vi "Turret_Homing.vi"(6 "Controller_Command":dbl, 7 "Turret_Motor_DefRef":T1={"DeviceStatus"={"status"=FALSE, "code"=0, "source"=""}, "Type"=enum."PWM", "PWM"={"PWM Channel"=enum."Invalid", "DeadBand"={"Name"="", "maxPositivePwm"=0, "minPositivePwm"=0, "centerPwm"=0, "maxNegativePwm"=0, "minNegativePwm"=0, "angularRange"=0}}, "CAN"={"Device Number"=0, "SetOutput VI Ref"=variant(enum8{"Percent VBus", "Current", "Speed", "Position", "Voltage"} enum."Percent VBus"), "GetOutput VI Ref"=variant(refnum<k1> refnum), "Enable VI Ref"=variant(dbl 12.0), "Disable VI Ref"=variant(enum8{"Percent VBus", "Speed", "Position", "Slave", "Unchanged / Invalid", "Voltage Compensation", "Current", "Motion Profile"} enum."Percent VBus"), "Data"=variant}, "Invert"=FALSE, "DIO PWM"={"PWM \"Enable\" Channel"=enum."Invalid", "DIOChannel"=enum."Invalid", "PWM Rate"=0.0}}, 8 "TurretManualHoming":bool, 9 "Reset":bool, 10 "Home_Position":dbl, 11 "MotorConfig":T6={"CAN Address"=0, "Invert"=FALSE, "InvertSensor"=FALSE, "Unit Conversion Factor"=0.0, "Brake Mode"=enum."Override to Brake", "Reverse Limt Switch Mode"=enum."Disabled", "Forward Limt Swith Mode"=enum."Disabled", "PWM Channel"=enum."Invalid", "Motor Controller Type"=enum."Talon SRX", "Peak Current (A)"=0, "Continuous Current (A)"=0, "Peak Duration (ms)"=0, "Current Limit Enable"=FALSE}) -> (1 "Motor_Output":dbl, 2 "Homing_State":T10, 3 "Turret_Motor_DefRef Out":T1={"DeviceStatus"={"status"=FALSE, "code"=0, "source"=""}, "Type"=enum."PWM", "PWM"={"PWM Channel"=enum."Invalid", "DeadBand"={"Name"="", "maxPositivePwm"=0, "minPositivePwm"=0, "centerPwm"=0, "maxNegativePwm"=0, "minNegativePwm"=0, "angularRange"=0}}, "CAN"={"Device Number"=0, "SetOutput VI Ref"=variant(enum8{"Percent VBus", "Current", "Speed", "Position", "Voltage"} enum."Percent VBus"), "GetOutput VI Ref"=variant(refnum<k1> refnum), "Enable VI Ref"=variant(dbl 12.0), "Disable VI Ref"=variant(enum8{"Percent VBus", "Speed", "Position", "Slave", "Unchanged / Invalid", "Voltage Compensation", "Current", "Motion Profile"} enum."Percent VBus"), "Data"=variant}, "Invert"=FALSE, "DIO PWM"={"PWM \"Enable\" Channel"=enum."Invalid", "DIOChannel"=enum."Invalid", "PWM Rate"=0.0}}, 5 "MotorConfigOut":T6={"CAN Address"=0, "Invert"=FALSE, "InvertSensor"=FALSE, "Unit Conversion Factor"=0.0, "Brake Mode"=enum."Override to Brake", "Reverse Limt Switch Mode"=enum."Disabled", "Forward Limt Swith Mode"=enum."Disabled", "PWM Channel"=enum."Invalid", "Motor Controller Type"=enum."Talon SRX", "Peak Current (A)"=0, "Continuous Current (A)"=0, "Peak Duration (ms)"=0, "Current Limit Enable"=FALSE})   [LabVIEW 2019]
uses:
  <vilib>/Rock Robotics/WPI/MotorControl/WPI_MotorControlDeviceRef.ctl
  <vilib>/Rock Robotics/WPI/MotorControl/WPI_MotorControlType.ctl
  <vilib>/Rock Robotics/SystemInterfaces/DIO/FPGA_DIOPWMChannel.ctl
  <vilib>/Rock Robotics/WPI/PWM/WPI_PWMDeadband.ctl
  <vilib>/Rock Robotics/SystemInterfaces/DIO/FPGA_DIOChannel.ctl
  ArgosLib/Config/ConfigComponents/TypeDefs/Config_Motor.ctl
  <vilib>/Rock Robotics/WPI/ThirdParty/Phoenix-LabVIEW/Motor Controller/Controls/CTRE_Phoenix_MotorControl_NeutralMode.ctl
  <vilib>/Rock Robotics/WPI/ThirdParty/Phoenix-LabVIEW/Motor Controller/Controls/CTRE_Phoenix_MotorControl_LimitSwitchNormal.ctl
  ArgosLib/Config/ConfigComponents/TypeDefs/Config_MotorCtrlType.ctl
  TypeDefs/Hood_Homing_State.ctl
  ArgosLib/Signal Processing/TypeDefs/EdgeDetector_Type.ctl
  <vilib>/Rock Robotics/WPI/ThirdParty/Phoenix-LabVIEW/Motor Controller/Controls/CTRE_Phoenix_MotorControl_FeedbackDevice.ctl
  TypeDefs/Read_or_Write.ctl
  584e72e6-e2ca-4219-9e99-eb915a757e0e.vi
  <vilib>/Rock Robotics/WPI/ThirdParty/Phoenix-LabVIEW/Motor Controller/Get/CTRE_Phoenix_MotorController_GetPulseWidthAll.vi
  <vilib>/Rock Robotics/WPI/ThirdParty/Phoenix-LabVIEW/Motor Controller/Get/CTRE_Phoenix_MotorController_GetSelectedSensorData.vi
  ArgosLib/ArgosLib.lvlib
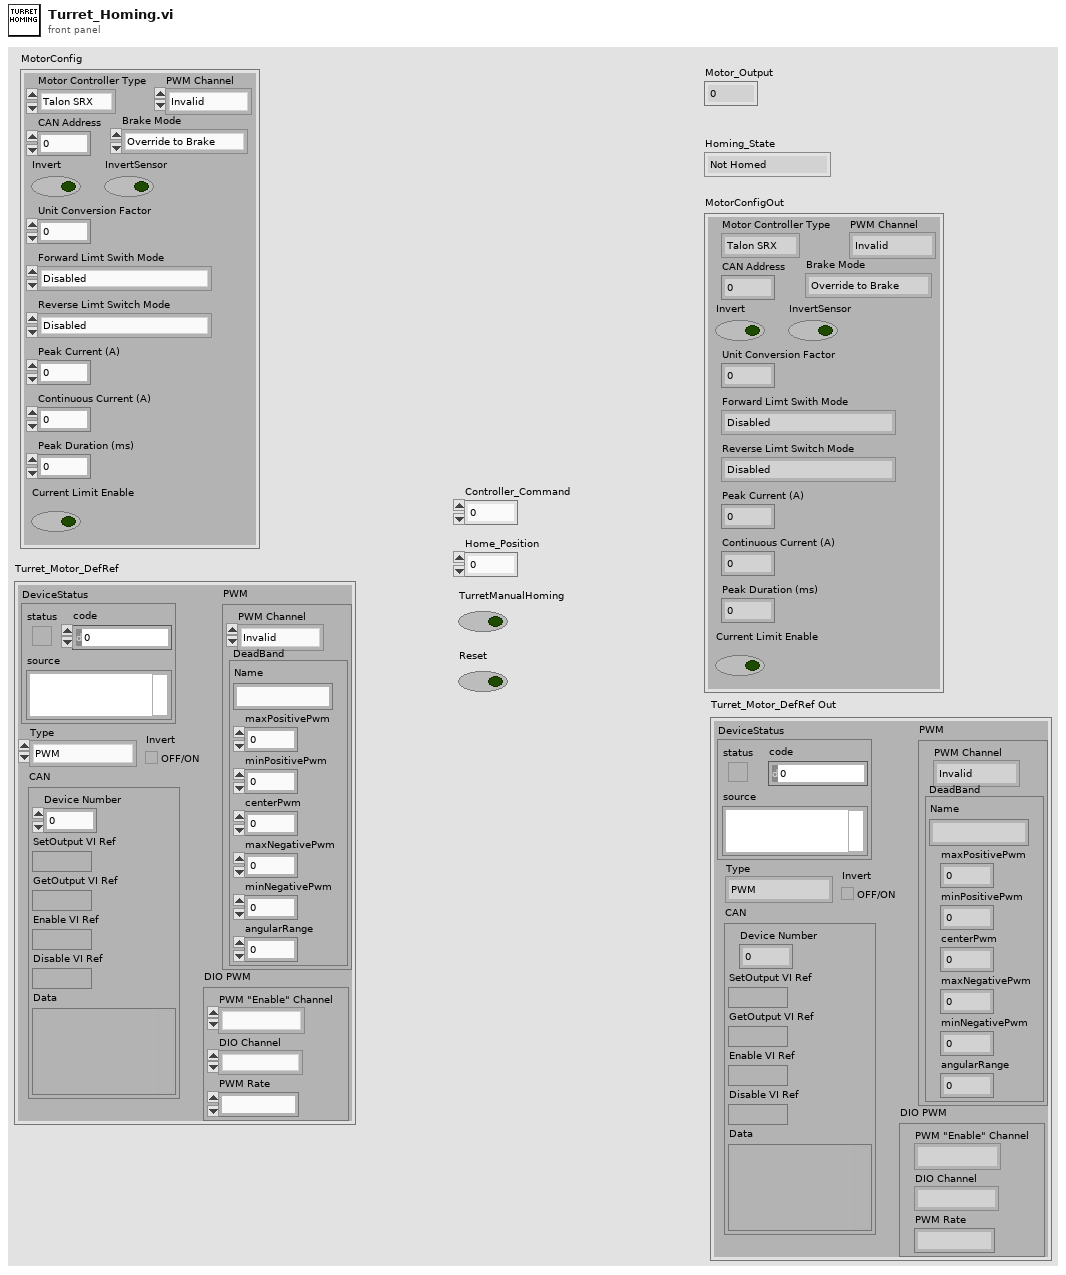
[diagram p1: front panel]
types:
  T1 = typedef "WPI_MotorControlDeviceRef.ctl" = cluster{"DeviceStatus":errorcluster, "Type":T2, "PWM":cluster{"PWM Channel":T3, "DeadBand":T4}, "CAN":cluster{"Device Number":u8, "SetOutput VI Ref":variant, "GetOutput VI Ref":variant, "Enable VI Ref":variant, "Disable VI Ref":variant, "Data":variant}, "Invert":bool, "DIO PWM":cluster{"PWM \"Enable\" Channel":T3, "DIOChannel":T5, "PWM Rate":dbl}}
  T2 = typedef "WPI_MotorControlType.ctl" = enum16{"PWM", "CAN", "DIO PWM"}
  T3 = typedef "FPGA_DIOPWMChannel.ctl" = enum8{"PWM 0", "PWM 1", "PWM 2", "PWM 3", "PWM 4", "PWM 5", "PWM 6", "PWM 7", "PWM 8", "PWM 9", "PWM MXP 0", "PWM MXP 1", "PWM MXP 2", "PWM MXP 3", "PWM MXP 4", "PWM MXP 5", "PWM MXP 6", "PWM MXP 7", "PWM MXP 8", "PWM MXP 9", "Invalid"}
  T4 = typedef "WPI_PWMDeadband.ctl" = cluster{"Name":string, "maxPositivePwm":i32, "minPositivePwm":i32, "centerPwm":i32, "maxNegativePwm":i32, "minNegativePwm":i32, "angularRange":u16}
  T5 = typedef "FPGA_DIOChannel.ctl" = enum8{"DIO 0", "DIO 1", "DIO 2", "DIO 3", "DIO 4", "DIO 5", "DIO 6", "DIO 7", "DIO 8", "DIO 9", "DIO MXP 0", "DIO MXP 1", "DIO MXP 2", "DIO MXP 3", "DIO MXP 4", "DIO MXP 5", "DIO MXP 6", "DIO MXP 7", "DIO MXP 8", "DIO MXP 9", "DIO MXP 10", "DIO MXP 11", "DIO MXP 12", "DIO MXP 13", "DIO MXP 14", "DIO MXP 15", "SPI Port CS1", "SPI Port CS2", "SPI Port CS3", "SPI Port MISO", "SPI Port MOSI", "Invalid"}
  T6 = typedef "ArgosLib.lvlib/Config_Motor.ctl" = cluster{"CAN Address":u8, "Invert":bool, "InvertSensor":bool, "Unit Conversion Factor":dbl, "Brake Mode":T7, "Reverse Limt Switch Mode":T8, "Forward Limt Swith Mode":T8, "PWM Channel":T3, "Motor Controller Type":T9, "Peak Current (A)":i32, "Continuous Current (A)":i32, "Peak Duration (ms)":i32, "Current Limit Enable":bool}
  T7 = typedef "CTRE_Phoenix_MotorControl_NeutralMode.ctl" = enum8{"EEPROMSetting", "Override to Coast", "Override to Brake"}
  T8 = typedef "CTRE_Phoenix_MotorControl_LimitSwitchNormal.ctl" = enum16{"Normally Open", "Normally Closed", "Disabled"}
  T9 = typedef "ArgosLib.lvlib/Config_MotorCtrlType.ctl" = enum16{"Disabled", "Talon SRX", "Talon SR", "Venom", "Spark MAX", "Falcon FX"}
  T10 = typedef "Hood_Homing_State.ctl" = enum16{"Not Homed", "Homing in Process", "Homing Failed", "Homing Completed"}
  T11 = typedef "ArgosLib.lvlib/EdgeDetector_Type.ctl" = enum16{"RisingEdge", "FallingEdge", "Both"}
  T12 = typedef "CTRE_Phoenix_MotorControl_FeedbackDevice.ctl" = i8
  T13 = typedef "Read_or_Write.ctl" = enum16{"Read", "Write"}
  T14 = typedef "CTRE_Phoenix_MotorControl_Faults.ctl" = cluster{"Under Voltage":bool, "Forward Limit Switch":bool, "Reverse Limit Switch":bool, "Forward Soft Limit":bool, "Reverse Soft Limit":bool, "Hardware Failure":bool, "Reset During Enable":bool, "Sensor Overflow":bool, "Sensor Out of Phase":bool, "Hardware ESD Reset":bool, "Remote Loss of Signal":bool}
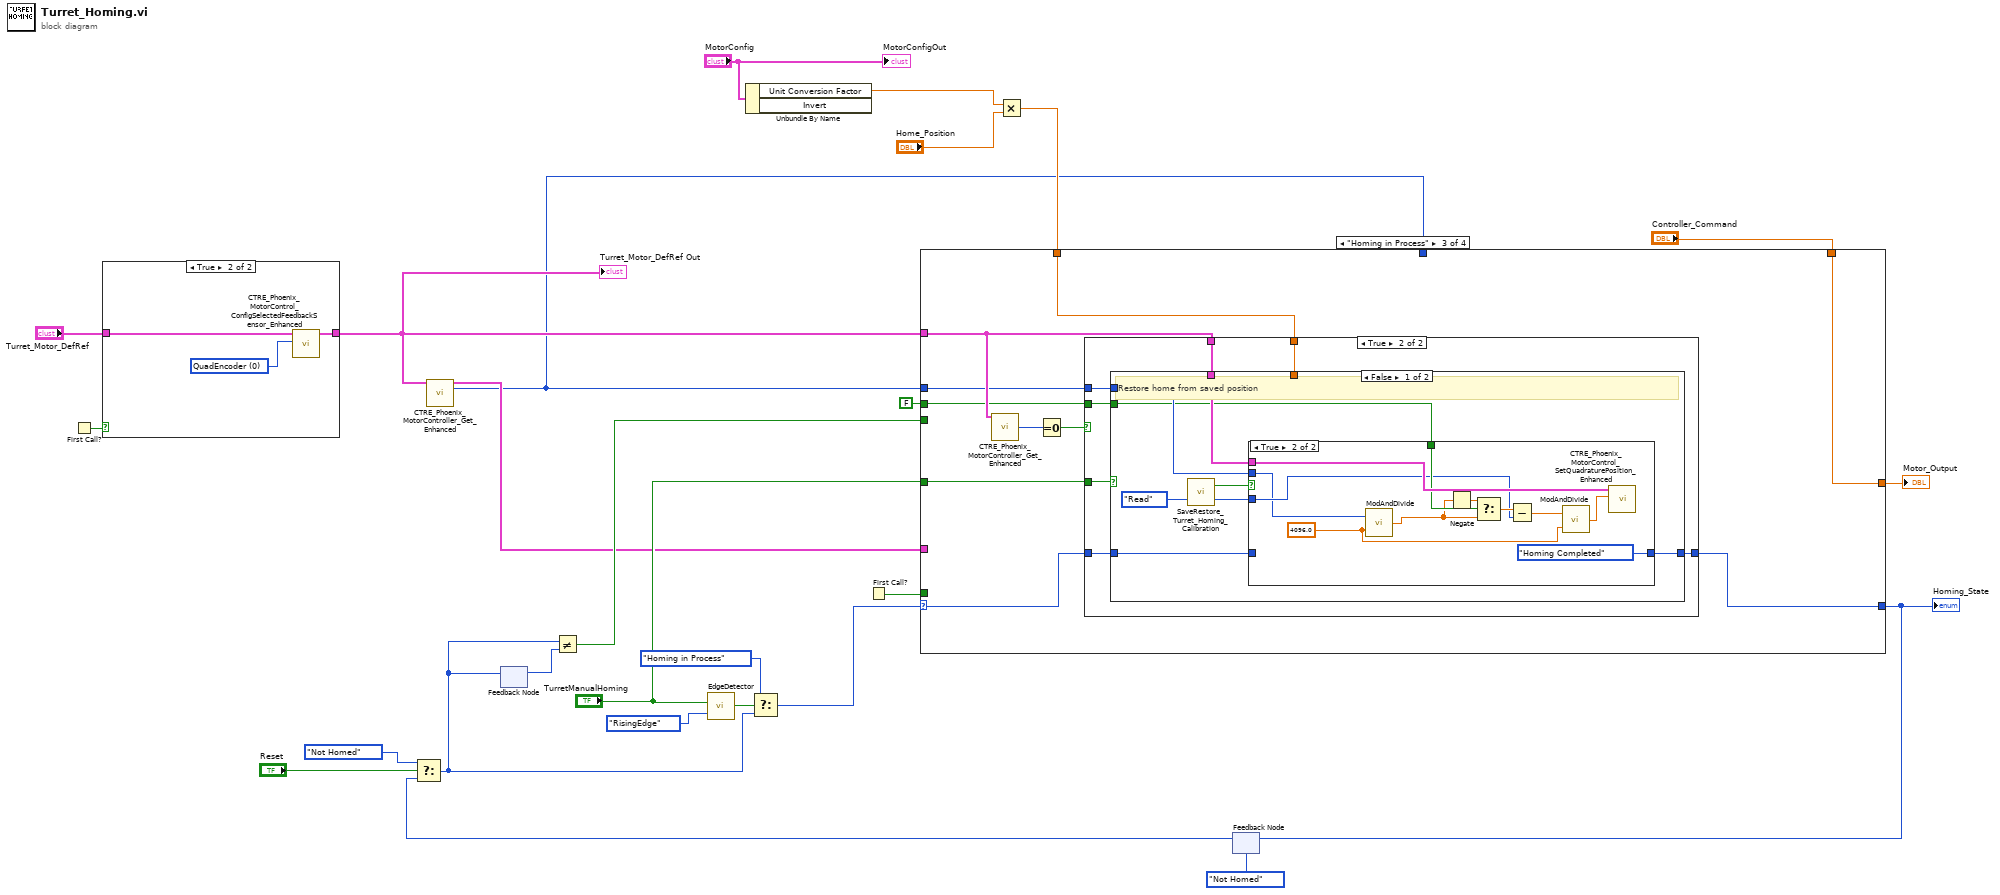
[diagram p0: block diagram]
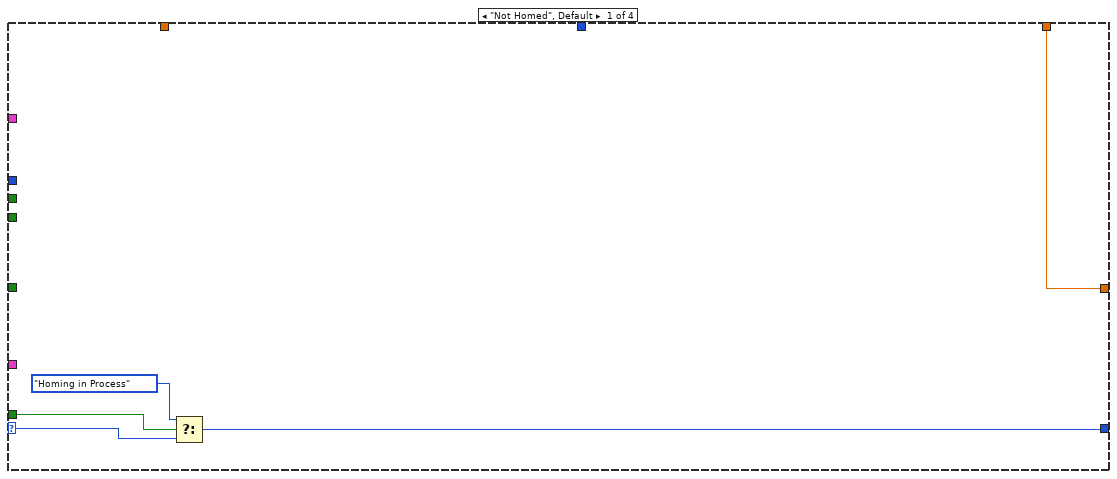
[diagram p3: hidden frame]
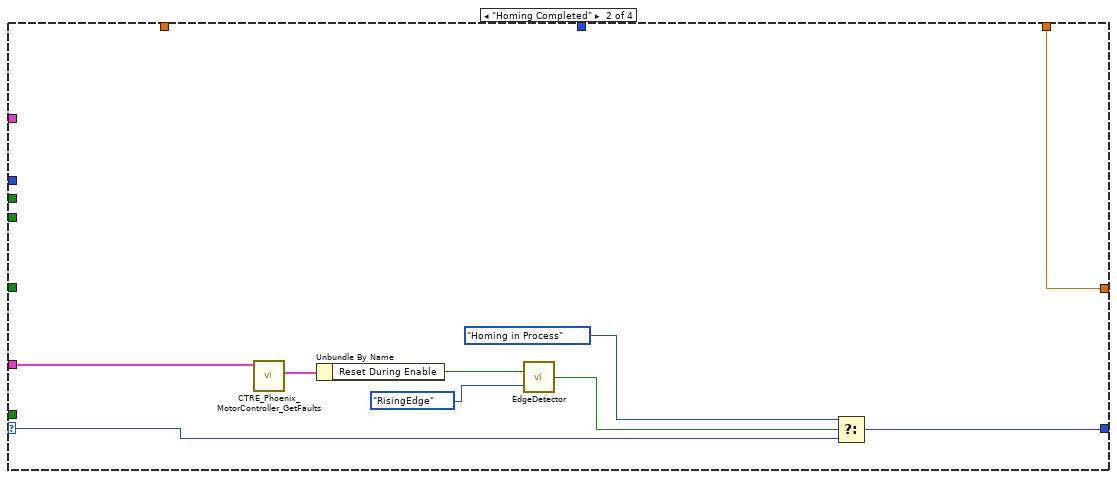
[diagram p4: hidden frame]
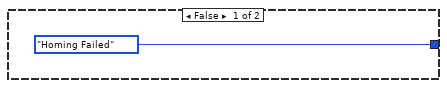
[diagram p6: hidden frame]
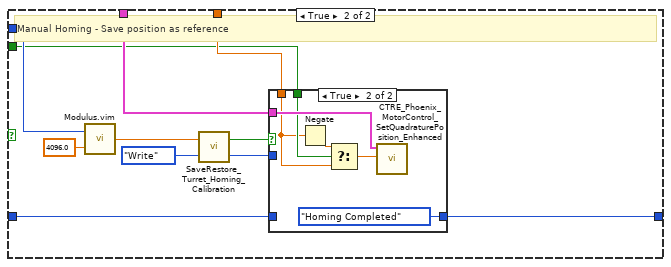
[diagram p7: hidden frame]
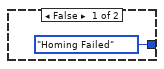
[diagram p8: hidden frame]
diagram:
  n1 = First Call?() -> (First Call?: T/F=w13:bool)
  n2 = case shown="True" w13 {
    tunnel: "Turret_Motor_DefRef" -> [w27 w30]
    tunnel: [w27 w28] -> w10
    frame False {
    }
    frame True {
      w29 = T12 0 items=["QuadEncoder"=0, "Analog"=2, "Tachometer"=4, "Pulse Width Encoded Position"=8, "Sensor Sum (S0 + S1)"=9, "Sensor Difference (D0 - D1)"=10, "Remote Source 0"=11, "Remote Source 1"=12, "Software Emulated"=15] ("Feedback Device")
      n3 = call <vilib>:"CTRE_Phoenix_MotorControl_ConfigSelectedFeedbackSensor_Enhanced.vi"("Feedback Device"=w29, "PhoenixMotorControlDevRef"=w30) -> ("PhoenixMotorControlDevRef"=w28:T1)  [unwired: 8 in, 1 out]
    }
  }
  "Turret_Motor_DefRef Out" <- w10
  n4 = call-poly <vilib>:"CTRE_Phoenix_MotorController_Get_Enhanced.vi"("PhoenixMotorControlDevRef"=w10) -> ("PhoenixMotorControlDevRef"=w7:T1, "Pulse Width Position"=w2:i32)  [unwired: 9 in, 4 out]
  n5 = feedback #1() -> (w22:T10)  [unwired: 1 in]
  n6 = call "EdgeDetector.vi"("DetectorType"=EdgeDetector_Type."RisingEdge", "Input"="TurretManualHoming") -> ("Edge"=w18:bool)
  n7 = Unbundle By Name("MotorConfig") -> ("Unit Conversion Factor"=w5:dbl)  [unwired: 1 out]
  n8 = First Call?() -> (First Call?: T/F=w6:bool)
  n9 = Multiply(x=w5, y="Home_Position") -> (x*y=w3:dbl)
  n10 = feedback #2(Hood_Homing_State."Not Homed") -> (w9:T10)
  n11 = Select(t=Hood_Homing_State."Not Homed", s="Reset", f=w9) -> (s? t:f=w17:T10)
  n12 = feedback-in #1(w17) -> ()
  n13 = Not Equal?(x=w17, y=w22) -> (x != y?=w21:bool)
  n14 = Select(t=Hood_Homing_State."Homing in Process", s=w18, f=w17) -> (s? t:f=w15:T10)
  n15 = case shown="\"Homing in Process\"" w15 {
    selector: w15 -> [w34 w36 w50 w101]
    tunnel: w6 -> [w32 _ _ _]
    tunnel: [w33 w40 w49 w101] -> w25
    tunnel: [w31 w44 w48 w102] -> w23
    tunnel: w21 -> [_ _ _ _]
    tunnel: w10 -> [_ _ w52 _]
    tunnel: "Controller_Command" -> [w31 w44 w48 w102]
    tunnel: "TurretManualHoming" -> [_ _ w47 _]
    tunnel: w2 -> [_ _ _ _]
    tunnel: w7 -> [_ w37 _ _]
    tunnel: w2 -> [_ _ w51 _]
    tunnel: w3 -> [_ _ w46 _]
    tunnel: FALSE ("Invert") -> [_ _ w45 _]
    frame "Not Homed", Default {
      n16 = Select(t=Hood_Homing_State."Homing in Process", s=w32, f=w34) -> (s? t:f=w33:T10)
    }
    frame "Homing Completed" {
      n17 = call <vilib>:"CTRE_Phoenix_MotorController_GetFaults.vi"("PhoenixMotorControlDevRef"=w37) -> ("Faults"=w42:T14)  [unwired: 8 in, 2 out]
      n18 = Unbundle By Name(w42) -> ("Reset During Enable"=w43:bool)
      n19 = call "EdgeDetector.vi"("DetectorType"=EdgeDetector_Type."RisingEdge", "Input"=w43) -> ("Edge"=w39:bool)
      n20 = Select(t=Hood_Homing_State."Homing in Process", s=w39, f=w36) -> (s? t:f=w40:T10)
    }
    frame "Homing in Process" {
      n21 = call-poly <vilib>:"CTRE_Phoenix_MotorController_Get_Enhanced.vi"("PhoenixMotorControlDevRef"=w52) -> ("Velocity (Raw Sensor Units per 100 ms)"=w54:i32)  [unwired: 11 in, 3 out]
      n22 = Equal To 0?(x=w54) -> (x = 0?=w53:bool)
      n23 = case shown="True" w53 {
        tunnel: w52 -> [_ w62]
        tunnel: w51 -> [_ w61]
        tunnel: w50 -> [w55 w60]
        tunnel: [w55 w59] -> w49
        tunnel: w47 -> [_ w58]
        tunnel: w46 -> [_ w57]
        tunnel: w45 -> [_ w56]
        frame False {
        }
        frame True {
          n24 = case shown="False" w58 {
            tunnel: w62 -> [w67 w89]
            tunnel: w61 -> [w66 w84]
            tunnel: w60 -> [w65 w90]
            tunnel: [w64 w88] -> w59
            tunnel: w57 -> [_ w87]
            tunnel: w56 -> [w63 w83]
            frame False {
              # "Restore home from saved position"
              n25 = call "SaveRestore_Turret_Homing_Calibration.vi"("ReadWrite_Mode"=Read_or_Write."Read") -> ("Turret_Home_Set"=w68:i32, "Load/Save_successful?"=w69:bool)  [unwired: 1 in]
              n26 = case shown="True" w69 {
                tunnel: w68 -> [_ w76]
                tunnel: w67 -> [_ w82]
                tunnel: w66 -> [_ w75]
                tunnel: w65 -> [_ _]
                tunnel: [Hood_Homing_State."Homing Failed" Hood_Homing_State."Homing Completed"] -> w64
                tunnel: w63 -> [_ w80]
                frame False {
                }
                frame True {
                  w73 = 4096.0 ("y")
                  n27 = call "ModAndDivide.vi"("y"=w73, "x"=w75) -> ("x%y ranged"=w78:dbl)
                  n28 = Negate(x=w78) -> (-x=w79:dbl)
                  n29 = Select(t=w79, s=w80, f=w78) -> (s? t:f=w77:dbl)
                  n30 = Subtract(x=w77, y=w76) -> (x-y=w74:dbl)
                  n31 = call "ModAndDivide.vi"("y"=w73, "x"=w74) -> ("x%y ranged"=w72:dbl)
                  n32 = call <vilib>:"CTRE_Phoenix_MotorControl_SetQuadraturePosition_Enhanced.vi"("New Position"=w72, "PhoenixMotorControlDevRef"=w82) -> ()  [unwired: 8 in, 2 out]
                }
              }
            }
            frame True {
              # "Manual Homing - Save position as reference"
              n33 = call "Modulus.vim"("y"=4096.0, "x"=w84) -> ("x%y"=w85:dbl)
              n34 = call "SaveRestore_Turret_Homing_Calibration.vi"("ReadWrite_Mode"=Read_or_Write."Write", "Turret_Offset (SensorUnits)"=w85) -> ("Turret_Home_Set"=w91:i32, "Load/Save_successful?"=w92:bool)
              n35 = case shown="True" w92 {
                tunnel: w91 -> [_ _]
                tunnel: w89 -> [_ w100]
                tunnel: w90 -> [_ _]
                tunnel: [Hood_Homing_State."Homing Failed" Hood_Homing_State."Homing Completed"] -> w88
                tunnel: w87 -> [_ w95]
                tunnel: w83 -> [_ w98]
                frame False {
                }
                frame True {
                  n36 = Negate(x=w95) -> (-x=w96:dbl)
                  n37 = Select(t=w96, s=w98, f=w95) -> (s? t:f=w97:dbl)
                  n38 = call <vilib>:"CTRE_Phoenix_MotorControl_SetQuadraturePosition_Enhanced.vi"("New Position"=w97, "PhoenixMotorControlDevRef"=w100) -> ()  [unwired: 8 in, 2 out]
                }
              }
            }
          }
        }
      }
    }
    frame "Homing Failed" {
    }
  }
  "Motor_Output" <- w23
  "Homing_State" <- w25
  n39 = feedback-in #2(w25) -> ()
  "MotorConfigOut" <- "MotorConfig"
